vi "Target Selection.vi"   [LabVIEW 2011]
uses:
  Robot Global Data.vi
types:
  T1 = typedef "WPI_JoystickDevRef.ctl" = cluster{"Device":T2}
  T2 = typedef "WPI_JoystickDeviceEnum.ctl" = enum16{"USB 1", "USB 2", "USB 3", "USB 4", "Kinect 1", "Kinect 2"}
  T3 = cluster{"Position":cluster{"X":dbl, "Y":dbl}, "Distance (ft)":dbl}[]
  T4 = typedef "WPI_JoystickButtonState.ctl" = cluster{"Button 1":bool, "Button 2":bool, "Button 3":bool, "Button 4":bool, "Button 5":bool, "Button 6":bool, "Button 7":bool, "Button 8":bool, "Button 9":bool, "Button 10":bool, "Button 11":bool, "Button 12":bool}
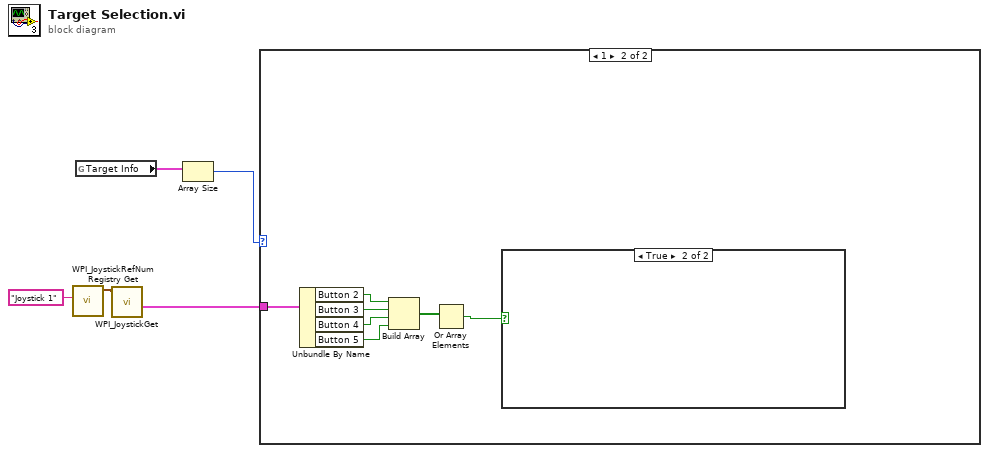
[diagram p0: block diagram]
diagram:
  n1 = call <vilib>:"WPI_JoystickRefNum Registry Get.vi"("refnum name"="Joystick 1") -> ("JoystickDevRef"=w4:T1)  [unwired: 9 in, 1 out]
  n2 = global read "Robot Global Data.vi" "Target Info"() -> (w1:T3)
  n3 = call <vilib>:"WPI_JoystickGet.vi"("JoystickDevRef"=w4) -> ("Buttons"=w2:T4)  [unwired: 4 in, 2 out]
  n4 = Array Size(array=w1) -> (size(s)=w3:i32)
  n5 = case shown="1" w3 {
    tunnel: w2 -> [_ w12]
    frame 0, Default {
    }
    frame 1 {
      n6 = Unbundle By Name(w12) -> ("Button 2"=w11:bool, "Button 3"=w10:bool, "Button 4"=w9:bool, "Button 5"=w8:bool)
      n7 = Build Array(w11, w10, w9, w8) -> (w7:bool[])
      n8 = Or Array Elements(Boolean array=w7) -> (logical OR=w6:bool)
      n9 = case shown="True" w6 {
        frame False {
        }
        frame True {
        }
      }
    }
  }
